vi "Test_LED.vi"   [LabVIEW 2016]
uses:
  <vilib>/NI_Real-Time Target Support.lvlib
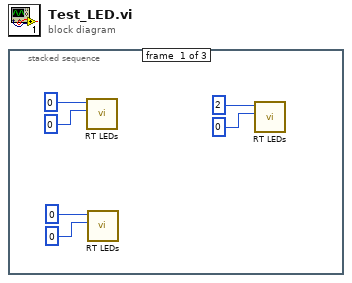
[diagram p0: block diagram]
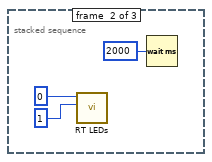
[diagram p2: hidden frame]
diagram:
  n1 = stacked-sequence {
    frame #0 {
      n2 = call <vilib>:"RT LEDs.vi"("State"=0, "LED Num"=0) -> ()  [unwired: 4 in, 2 out]
      n3 = call <vilib>:"RT LEDs.vi"("State"=0, "LED Num"=0) -> ()  [unwired: 4 in, 2 out]
      n4 = call <vilib>:"RT LEDs.vi"("State"=0, "LED Num"=2) -> ()  [unwired: 4 in, 2 out]
    }
    frame #1 {
      n5 = call <vilib>:"RT LEDs.vi"("State"=1, "LED Num"=0) -> ()  [unwired: 4 in, 2 out]
      n6 = Wait (ms)(milliseconds to wait=u32 2000) -> ()  [unwired: 1 out]
    }
    frame #2 {
    }
  }
